vi "SVFA Power Spectral Density Subset (1 Ch).vi"(0 "scaled signal [EU]":waveform(dbl)={"t0"=timestamp(0 s since 1904-01-01), "dt"=1e-05, "Y"=[]}, 2 "window":T7=1 items=["None"=0, "Hanning"=1, "Hamming"=2, "Blackman-Harris"=3, "Exact Blackman"=4, "Blackman"=5, "Flat Top"=6, "4 Term B-Harris "=7, "7 Term B-Harris"=8, "Low Sidelobe"=9, "Force"=64, "Exponential"=65, "Blackman Nuttall"=11, "Triangle"=30, "Bartlett-Hanning"=31, "Bohman"=32, "Parzen"=33, "Welch"=34, "Kaiser"=60, "Dolph-Chebyshev"=61, "Gaussian"=62], 3 "frequency range":T9={"start frequency"=1000.0, "stop frequency"=5000.0} {"stop frequency" min=0.0 format="%.2f"; "start frequency" min=0.0 format="%.2f"}, 4 "dB On (F)":bool, 5 "error in (no error)":errorcluster, 6 "desired units":enum16{"EU^2 / Hz", "EU / sqrt(Hz)"}(ring), 7 "averaging parameters":T8={"averaging mode"=enum."No averaging", "weighting mode"=enum."Exponential", "number of averages"=10, "linear mode"=enum."One shot"} {"number of averages" min=1 step=1}, 9 "restart averaging (F)":bool) -> (11 "averaging done":bool, 13 "averages completed":dbl, 14 "power spectral density [EU^2 rms / Hz]":cluster{"f0":dbl, "df":dbl, "magnitude":dbl[]}={"f0"=nan, "df"=inf, "magnitude"=[]} {"magnitude" format="%.2p"; "df" format="%.2p"; "f0" format="%.2p"}, 15 "unit label":string, 18 "spectrum info":T1={"channel name"="", "description"="", "x-axis units"=1, "spectral info"={"spectrum type"=enum."Power [Magnitude^2]", "linear/dB"=enum."linear", "window"=0, "window size"=0, "FFT size"=0}, "engineering units"=0, "custom label"="", "dB reference [EU]"=0.0, "peak units"=enum."rms", "weighting filter"=0, "spectral density?"=FALSE, "unit label"="", "spectrum skewed?"=FALSE, "complimentary spectrum units"=enum."none"} {"x-axis units" items=["Time (s)"=0, "Frequency-CB (Hz)"=1, "Frequency-CPB (Hz)"=1248, "Frequency-Arbitrary (Hz)"=2357, "Quefrency (s)"=2, "Revolutions (rev)"=3, "Order"=4, "Speed (RPM)"=11, "Speed (rad/s)"=21, "Index"=65535]; "weighting filter" items=["Linear", "A-weighting", "B-weighting", "C-weighting", "ITU-R 468-4", "Dolby", "CCITT", "C-message", "Wb", "Wc", "Wd", "We", "Wf", "Wh", "Wj", "Wk", "Wm", "AES17 20 kHz lowpass", "AES17 40 kHz lowpass", "AES17 20 kHz highpass", "AES17 40 kHz highpass"]; "dB reference [EU]" format="%.2f"; "engineering units" items=["custom..."=0, "V"=1, "A"=21, "C"=30, "pC"=31, "s"=32, "-"=29, "Pa"=2, "N"=20, "g"=3, "m/s^2"=4, "m/s"=5, "m"=6, "mm/s"=12, "mm"=13, "micron/s"=14, "micron"=15, "in/s^2"=7, "in/s"=8, "in"=9, "mil/s"=10, "mil"=11, "rad/s^2"=16, "rad/s"=17, "rad"=18, "deg/s^2"=26, "deg/s"=27, "deg"=28, "RPM"=22, "cycle/s^2"=23, "Hz"=24, "cycle"=25, "strain"=19]; "spectral info"."window" items=["None "=0, "Hanning"=1, "Hamming"=2, "Blackman-Harris"=3, "Exact Blackman"=4, "Blackman"=5, "Flat Top"=6, "4 Term B-Harris "=7, "7 Term B-Harris"=8, "Low Sidelobe"=9, "Force - Exponential"=10, "Gaussian"=62]}, 19 "error out":errorcluster)   [LabVIEW 2017]
doc: "Computes a subset of the power spectral density of <B>scaled signal [EU]</B>. The subset is defined by <B>frequency range</B>. Each block of data corresponds to a single FFT block and has to be passed individually to this VI. Wire data to the <B>scaled signal [EU]</B> input to determine the polymorphic instance to use or manually select the instance."
uses:
  <vilib>/addons/_NISVFA/_Shared subVIs/Controls/svc_Window.ctl
  <vilib>/addons/_NISVFA/_Shared subVIs/Controls/svc_Spectrum Info.ctl
  <vilib>/addons/_NISVFA/_Shared subVIs/Controls/svc_X-Axis Units.ctl
  <vilib>/addons/_NISVFA/_Shared subVIs/Controls/svc_Spectrum Type.ctl
  <vilib>/addons/_NISVFA/_Shared subVIs/Controls/svc_Engineering Units Text Ring.ctl
  <vilib>/addons/_NISVFA/_Shared subVIs/Controls/svc_Weighting Filter Text Ring.ctl
  <vilib>/addons/_NISVFA/_Shared subVIs/Controls/svc_Complimentary Spectrum Units.ctl
  <vilib>/addons/_NISVFA/_Spectrum Processing/SVFA Unit Conversion (1 Ch).vi
  <vilib>/addons/_NISVFA/_Shared subVIs/Windowing/svfa_Scaled Time Domain Window (Array).vi
  <vilib>/addons/_NISVFA/_Shared subVIs/Common/svc_Get SV Channel Info.vi
  <vilib>/addons/_NISVFA/_Shared subVIs/Common/svc_Spectrum Units.vi
  <vilib>/addons/_NISVFA/_Shared subVIs/Spectrum Averaging/svfa_Reset Averaging State Info.vi
  <vilib>/addons/_NISVFA/_Shared subVIs/Spectrum Averaging/svfa_Average Array with Avg Checks (complex) No State.vi
  <vilib>/addons/_NISVFA/_Shared subVIs/Common/svc_Complex to Mag2 Array.vi
  <vilib>/addons/_NISVFA/_Shared subVIs/Spectrum Averaging/svfa_Average Array with Avg Checks (real) No State.vi
  <vilib>/addons/_NISVFA/_Spectrum Processing/subVIs/svfa_Conversion Utility (spectrum info).vi
  <vilib>/Analysis/4window.llb/Force Window.vi
  <vilib>/Analysis/4window.llb/Force Window (DBL).vi
  <vilib>/Analysis/4window.llb/Exponential Window.vi
  <vilib>/Analysis/4window.llb/Exponential Window (DBL).vi
  <vilib>/addons/_NISVFA/_Shared subVIs/Spectrum Averaging/svfa_Average Array (complex) No State.vi
  <vilib>/addons/_NISVFA/_Shared subVIs/Spectrum Averaging/svfa_Average Array (real) No State.vi
  <vilib>/addons/_NISVFA/_Spectrum Processing/subVIs/svfa_Peak to RMS to Peak2Peak.vi
  <vilib>/addons/_NISVFA/_Spectrum Processing/subVIs/svfa_Mag to Mag2.vi
  <vilib>/addons/_NISVFA/_Spectrum Processing/subVIs/svfa_Linear to dB.vi
  <vilib>/addons/_NISVFA/_Spectrum Processing/subVIs/svfa_dBrefA to dBrefB.vi
  <vilib>/addons/_NISVFA/_Spectrum Processing/subVIs/svfa_Spectrum to Spectral Density.vi
  <vilib>/addons/_NISVFA/_Shared subVIs/Spectrum Averaging/svfa_No Average Array (complex).vi
  <vilib>/addons/_NISVFA/_Shared subVIs/Spectrum Averaging/svfa_Average Array (complex).vi
  <vilib>/addons/_NISVFA/_Shared subVIs/Spectrum Averaging/svfa_No Average Array (real).vi
  <vilib>/addons/_NISVFA/_Shared subVIs/Spectrum Averaging/svfa_Average Array (real).vi
  <vilib>/addons/_NISVFA/_Shared subVIs/Spectrum Averaging/svfa_Peak Hold Array.vi
  <vilib>/addons/_NISVFA/_Shared subVIs/Common/svc_Get Weighting Enum and Labels.vi
  <vilib>/addons/_NISVFA/_Shared subVIs/Common/svc_Unit Label Lexical Class.vi
  <vilib>/addons/_NISVFA/_Shared subVIs/Common/svc_Engineering Units to Unit Label.vi
  <vilib>/addons/_NISVFA/_Shared subVIs/Common/svc_Format Value (DBL).vi
  <vilib>/addons/_NISVFA/_Shared subVIs/Common/svc_Window Parameters.vi
  <vilib>/addons/_NISVFA/_Shared subVIs/Common/svc_Channel Info to Spectrum Info.vi
  <vilib>/addons/_NISVFA/_Shared subVIs/Common/svc_Unit Label to Engineering Units.vi
  <vilib>/Utility/error.llb/Error Cluster From Error Code.vi
  <vilib>/Analysis/0measdsp.llb/Scaled Time Domain Window.vi
  <vilib>/Analysis/0measdsp.llb/Scaled Time Domain Window (DBL).vi
  <vilib>/addons/_NISVFA/_Spectrum Processing/subVIs/svfa_Spectrum Info Window to windowTd Type Def.vi
  <vilib>/addons/_NISVFA/_Shared subVIs/Common/svc_Get Window Info.vi
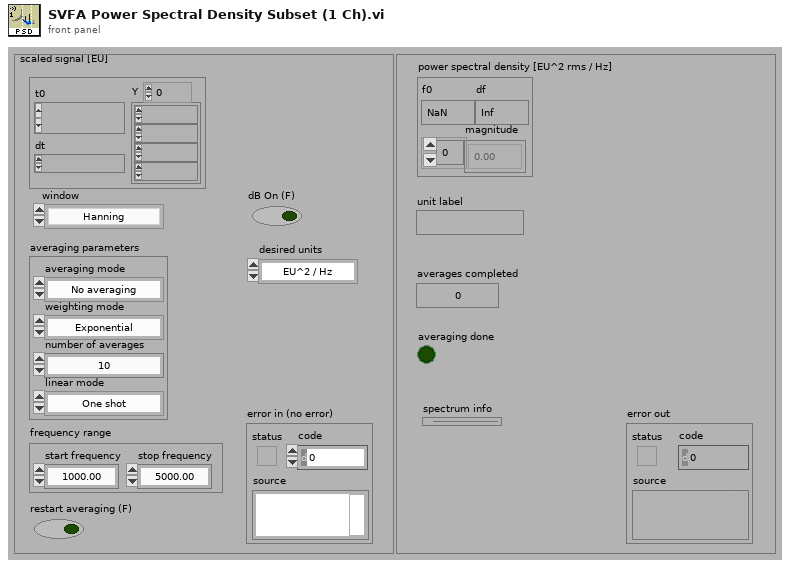
[diagram p1: front panel]
types:
  T1 = typedef "svc_Spectrum Info.ctl" = cluster{"channel name":string, "description":string, "x-axis units":T2, "spectral info":cluster{"spectrum type":T3, "linear/dB":enum16{"linear", "dB"}, "window":u16, "window size":i32, "FFT size":i32}, "engineering units":T4, "custom label":string, "dB reference [EU]":dbl, "peak units":enum16{"rms", "peak", "peak-peak"}, "weighting filter":T5, "spectral density?":bool, "unit label":string, "spectrum skewed?":bool, "complimentary spectrum units":T6}
  T2 = typedef "svc_X-Axis Units.ctl" = u16
  T3 = typedef "svc_Spectrum Type.ctl" = enum16{"FFT Spectrum [complex]", "Amplitude [Magnitude]", "Power [Magnitude^2]", "Cross Spectrum [complex]", "Frequency Response [Complex]"}
  T4 = typedef "svc_Engineering Units Text Ring.ctl" = u16
  T5 = typedef "svc_Weighting Filter Text Ring.ctl" = u16
  T6 = typedef "svc_Complimentary Spectrum Units.ctl" = enum16{"none", "radians", "degrees", "cycles", "imaginary"}
  T7 = typedef "svc_Window.ctl" = u32
  T8 = cluster{"averaging mode":enum16{"No averaging", "Vector averaging", "RMS averaging", "Peak hold"}, "weighting mode":enum16{"Linear", "Exponential"}, "number of averages":u32, "linear mode":enum16{"One shot", "Auto restart"}}
  T9 = cluster{"start frequency":dbl, "stop frequency":dbl}
  T10 = cluster{"linear/dB":enum16{"no change", "linear", "dB"}, "dB reference (0: no change)":dbl, "power/magnitude":enum16{"no change", "power", "magnitude"}, "view":enum16{"no change", "rms", "peak", "peak-peak"}}
  T11 = enum16{"Restart processing", "Continue processing", "Skip processing"}
  T12 = enum16{"no change", "spectrum", "spectral density"}
  T13 = enum16{"No averaging", "Vector averaging", "RMS averaging", "Peak hold"}
  T14 = cluster{"complex FFT":cdb[], "real FFT":dbl[], "f0":dbl, "df":dbl, "averages completed":dbl, "averaging parameters":cluster{"averaging mode":enum16{"No averaging", "Vector averaging", "RMS averaging", "Peak hold"}, "weighting mode":enum16{"Linear", "Exponential"}, "number of averages":u32, "linear mode":enum16{"One shot", "Auto restart"}}}
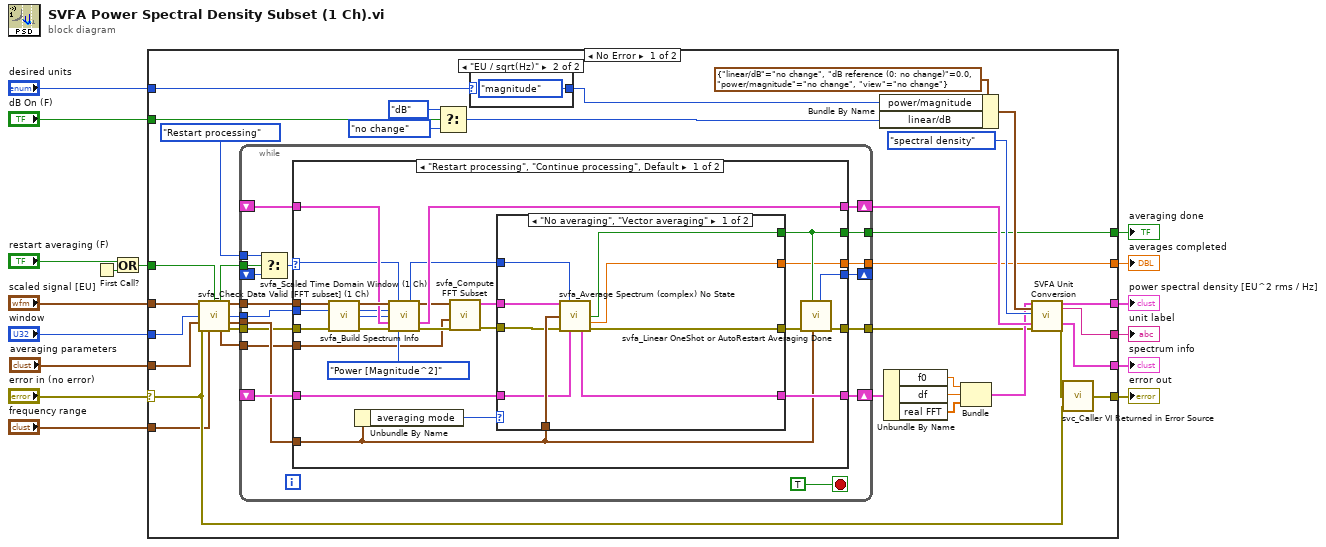
[diagram p0: block diagram]
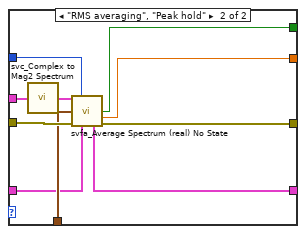
[diagram p2: hidden frame]
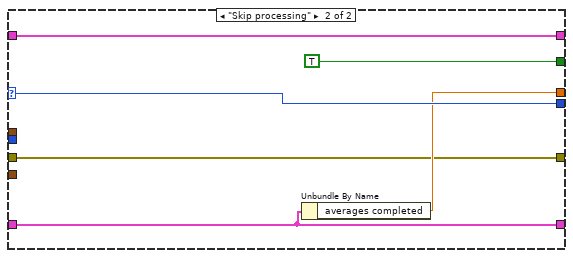
[diagram p3: hidden frame]
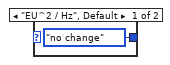
[diagram p4: hidden frame]
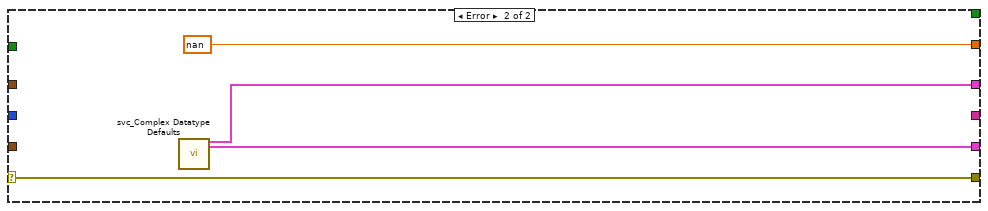
[diagram p5: hidden frame]
diagram:
  n1 = First Call?() -> (First Call?: T/F=w3:bool)
  n2 = Or(x="restart averaging (F)", y=w3) -> (x .or. y?=w2:bool)
  n3 = case shown="No Error" "error in (no error)" {
    selector: "error in (no error)" -> [w41 w127]
    tunnel: w2 -> [w46 _]
    tunnel: [w17 nan ("Averaged So-far")] -> w15
    tunnel: [w18 _] -> w14
    tunnel: [w48 w125] -> w9
    tunnel: [w42 w127] -> w13
    tunnel: "averaging parameters" -> [w45 _]
    tunnel: "frequency range" -> [w28 _]
    tunnel: "scaled signal [EU]" -> [w51 _]
    tunnel: "window" -> [w44 _]
    tunnel: "dB On (F)" -> [w47 _]
    tunnel: [w49 _] -> w4
    tunnel: "desired units" -> [w52 _]
    tunnel: [w50 w124] -> w5
    frame No Error {
      n4 = call <vilib>:"svfa_Check Data Valid [FFT subset] (1 Ch).vi"("signal"=w51, "restart averaging (F)"=w46, "window"=w44, "averaging parameters"=w45, "error in (no error)"=w41, "frequency range in"=w28) -> ("restart averaging"=w22:bool, "dup signal"=w23:waveform(dbl), "window"=w24:u16, "dup averaging parameters"=w25:T8, "frequency range out"=w27:T9, "error out"=w26:errorcluster)  [unwired: 4 in]
      n5 = while {
        shift-left: _ -> [w61]
        shift-right: [w62] -> w30
        tunnel: [w68] -> w17
        tunnel: [w69] -> w18
        tunnel: [w70] -> w19
        tunnel: w23 -> [w67]
        tunnel: w24 -> [w66]
        shift-right: [w64] -> w21
        shift-left: _ -> [w63]
        shift-right: [w60] -> _
        shift-left: _ -> [w59]
        tunnel: w25 -> [w57]
        tunnel: w26 -> [w56]
        tunnel: w22 -> [w55]
        tunnel: T11."Restart processing" ("t") -> [w54]
        tunnel: w27 -> [w53]
        stop <- TRUE stop-if-true
        n6 = Select(t=w54, s=w55, f=w59) -> (s? t:f=w58:T11)
        n7 = case shown="\"Restart processing\", \"Continue processing\", Default" w58 {
          selector: w58 -> [w73 w120]
          tunnel: w57 -> [w88 _]
          tunnel: [w79 w116] -> w64
          tunnel: [w95 w119] -> w62
          tunnel: [w87 w117] -> w70
          tunnel: [w92 TRUE ("averaging done?")] -> w69
          tunnel: [w91 w118] -> w68
          tunnel: w67 -> [w93 _]
          tunnel: w63 -> [w78 w116]
          tunnel: w61 -> [w86 w119]
          tunnel: [w89 w120] -> w60
          tunnel: w66 -> [w90 _]
          tunnel: w56 -> [w72 w117]
          tunnel: w53 -> [w71 _]
          frame "Restart processing", "Continue processing", Default {
            n8 = call <vilib>:"svfa_Scaled Time Domain Window (1 Ch).vi"("Signal in [X]"=w93, "window"=w90, "error in"=w72) -> ("Windowed Waveform"=w84:waveform(dbl), "dup window"=w77:T7, "window length"=w76:i32, "error out"=w80:errorcluster)  [unwired: 7 in, 2 out]
            n9 = Unbundle By Name(w88) -> ("averaging mode"=w96:T13)
            n10 = call <vilib>:"svfa_Build Spectrum Info.vi"("scaled signal [EU]"=w84, "processing control"=w73, "window"=w77, "window size"=w76, "spectrum info in"=w78, "error in (no error)"=w80, "spectrum type"=svc_Spectrum_Type."Power [Magnitude^2]" ("spectrum type 2")) -> ("dup processing control"=w75:T11, "dup scaled signal [EU]"=w74:waveform(dbl), "spectrum info out"=w79:T1, "error out"=w85:errorcluster)  [unwired: 5 in]
            n11 = call <vilib>:"svfa_Compute FFT Subset.vi"("error in (no error)"=w85, "frequency range"=w71, "windowed signal"=w74) -> ("error out"=w82:errorcluster, "FFT spectrum [Vrms]"=w81:cluster{"f0":dbl, "df":dbl, "spectrum":cdb[]})  [unwired: 7 in]
            n12 = case shown="\"No averaging\", \"Vector averaging\"" w96 {
              tunnel: w88 -> [w104 w109]
              tunnel: [w97 w106] -> w95
              tunnel: [w102 w113] -> w94
              tunnel: w81 -> [w105 w111]
              tunnel: w82 -> [w103 w115]
              tunnel: w75 -> [w99 w108]
              tunnel: [w100 w112] -> w91
              tunnel: w86 -> [w98 w107]
              tunnel: [w101 w114] -> w92
              frame "No averaging", "Vector averaging" {
                n13 = call <vilib>:"svfa_Average Spectrum (complex) No State.vi"("spectrum"=w105, "processing control"=w99, "averaging parameters"=w104, "error in (no error)"=w103, "averaging state info in"=w98) -> ("averaging done"=w101:bool, "averages completed"=w100:dbl, "averaging state info out"=w97:T14, "error out"=w102:errorcluster)  [unwired: 5 in, 2 out]
              }
              frame "RMS averaging", "Peak hold" {
                n14 = call <vilib>:"svc_Complex to Mag2 Spectrum.vi"("complex spectrum"=w111) -> ("power spectrum"=w110:cluster{"f0":dbl, "df":dbl, "spectrum":dbl[]})  [unwired: 4 in]
                n15 = call <vilib>:"svfa_Average Spectrum (real) No State.vi"("spectrum"=w110, "processing control"=w108, "averaging parameters"=w109, "error in (no error)"=w115, "averaging state info in"=w107) -> ("averaging done"=w114:bool, "averages completed"=w112:dbl, "averaging state info out"=w106:T14, "error out"=w113:errorcluster)  [unwired: 5 in, 2 out]
              }
            }
            n16 = call <vilib>:"svfa_Linear OneShot or AutoRestart Averaging Done.vi"("averaging parameters"=w88, "averaging done"=w92, "error in (no error)"=w94) -> ("error out"=w87:errorcluster, "processing control"=w89:T11)  [unwired: 7 in]
          }
          frame "Skip processing" {
            n17 = Unbundle By Name(w119) -> ("averages completed"=w118:dbl)
          }
        }
      }
      n18 = Select(t=enum16{"no change", "linear", "dB"}."dB" ("linear/dB"), s=w47, f=enum16{"no change", "linear", "dB"}."no change" ("linear/dB")) -> (s? t:f=w38:enum16{"no change", "linear", "dB"})
      n19 = case shown="\"EU / sqrt(Hz)\"" w52 {
        tunnel: [enum16{"no change", "power", "magnitude"}."no change" ("power/magnitude") enum16{"no change", "power", "magnitude"}."magnitude" ("power/magnitude")] -> w40
        frame "EU^2 / Hz", Default {
        }
        frame "EU / sqrt(Hz)" {
        }
      }
      n20 = Bundle By Name(cluster=T10 {"linear/dB"=enum."no change", "dB reference (0: no change)"=0.0, "power/magnitude"=enum."no change", "view"=enum."no change"} ("desired scaling"), "power/magnitude"=w40, "linear/dB"=w38) -> (w36:T10)
      n21 = Unbundle By Name(w30) -> ("f0"=w33:dbl, "df"=w32:dbl, "real FFT"=w31:dbl[])
      n22 = Bundle("f0"=w33, "df"=w32, "real FFT"=w31) -> (w20:cluster{"f0":dbl, "df":dbl, "real FFT":dbl[]})  [unwired: 1 in]
      n23 = call-poly <vilib>:"SVFA Unit Conversion.vi"("spectrum"=w20, "desired scaling"=w36, "spectral density desired"=T12."spectral density", "spectrum info in"=w21, "error in (no error)"=w19) -> ("converted spectrum"=w48:cluster{"x0":dbl, "dx":dbl, "magnitude":dbl[]}, "unit label"=w49:string, "spectrum info out"=w50:T1, "error out"=w43:errorcluster)  [unwired: 11 in]
      n24 = call <vilib>:"svc_Caller VI Returned in Error Source.vi"("warning input to caller"=w41, "error in (no error)"=w43) -> ("error out"=w42:errorcluster)  [unwired: 3 in]
    }
    frame Error {
      n25 = call <vilib>:"svc_Complex Datatype Defaults.vi"() -> ("empty spectrum"=w125:cluster{"f0":dbl, "df":dbl, "magnitude":dbl[]}, "dead spectrum info"=w124:T1)  [unwired: 11 in, 7 out]
    }
  }
  "averages completed" <- w15
  "averaging done" <- w14
  "error out" <- w13
  "power spectral density [EU^2 rms / Hz]" <- w9
  "unit label" <- w4
  "spectrum info" <- w5
